vi "1L08-num1D-vers-max_decimales.vi"(1 "num. déc. (1D)":dbl[](array[numeric])) -> (0 "Max déc.":i32)   [LabVIEW 2010, in "lv_01.lvlib"]
uses:
  lv_01.lvlib
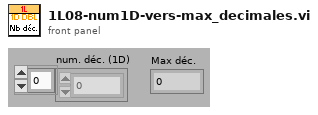
[diagram p1: front panel]
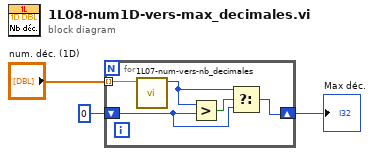
[diagram p0: block diagram]
diagram:
  n1 = for {
    tunnel: "num. déc. (1D)" -> [w8] mode=indexing
    shift-right: [w4] -> w3
    shift-left: 0 -> [w5]
    n2 = call "1L07-num-vers-nb_decimales.vi"("nombre"=w8) -> ("nb dec."=w6:i32)  [unwired: 10 in]
    n3 = Greater?(x=w6, y=w5) -> (0:w7:bool)
    n4 = Select(t=w6, s=w7, f=w5) -> (s? t:f=w4:i32)
  }
  "Max déc." <- w3
